vi "Adam Asma Yeni Kelime (SubVI).vi"(11 "Kelime":string) -> (1 "Bulunacak":string, 2 "Görüntülenecek":string, 3 "Aranacak":string)   [LabVIEW 8.6]
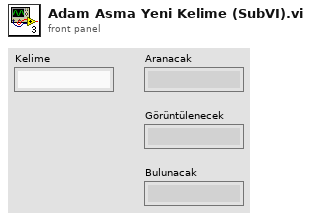
[diagram p1: front panel]
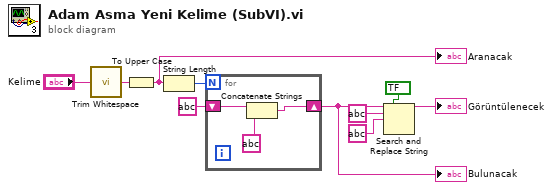
[diagram p0: block diagram]
diagram:
  n1 = call <vilib>:"Trim Whitespace.vi"("string"="Kelime") -> ("trimmed string"=w8:string)  [unwired: 1 in]
  n2 = To Upper Case(1:w8) -> (0:w9:string)
  "Aranacak" <- w9
  n3 = String Length(string=w9) -> (length=w1:i32)
  n4 = for {
    N: w1 -> [_]
    shift-right: [w11] -> w10
    shift-left: string ? ("Kelime") -> [w13]
    n5 = Concatenate Strings(w13, string ? ("Kelime")) -> (w11:string)
  }
  "Bulunacak" <- w10
  n6 = Search and Replace String(replace all?=bool ? ("replace all? (F)"), input string=w10, search string=string ?, replace string=string ? ("replace string (\"\")")) -> (result string=→"Görüntülenecek":string)  [unwired: 4 in, 3 out]
